vi "Send Write.vi"(8 "error in":errorcluster, 10 "Write":bool, 11 "MBs":refnum<class "Modbus Master CR.lvclass">[](array[class])) -> (0 "error out":errorcluster, 3 "MBs out":refnum<class "Modbus Master CR.lvclass">[](array[class]))   [LabVIEW 2021, in "Modbus Master CR.lvclass"]
uses:
  Modbus Master CR.lvclass
  Modbus Master CR.lvclass/Modbus Master CR.ctl
  <vilib>/Utility/error.llb/Clear Errors.vi
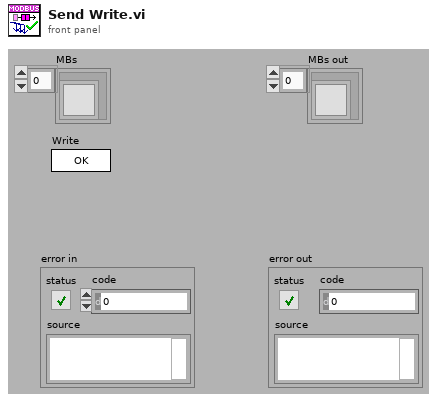
[diagram p1: front panel]
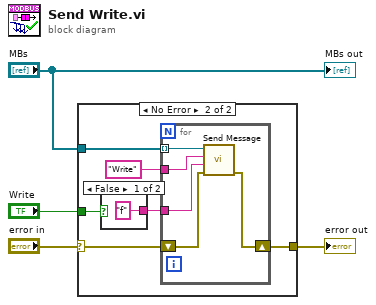
[diagram p0: block diagram]
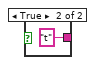
[diagram p3: hidden frame]
diagram:
  n1 = case shown="No Error" "error in" {
    selector: "error in" -> [w5 w11]
    tunnel: [w5 w8] -> w4
    tunnel: "MBs" -> [_ w6]
    tunnel: "Write" -> [_ w7]
    frame Error {
    }
    frame No Error {
      n2 = case shown="False" w7 {
        tunnel: ["f" ("Message") "t" ("Message")] -> w9
        frame False {
        }
        frame True {
        }
      }
      n3 = for {
        tunnel: "Write" ("Message") -> [w16]
        tunnel: w9 -> [w15]
        shift-right: [w14] -> w8
        shift-left: w11 -> [w13]
        tunnel: w6 -> [w12] mode=indexing
        n4 = call "Send Message.vi"("error in (no error)"=w13, "Message Data"=w15, "Message"=w16, "MB in"=w12) -> ("error out"=w14:errorcluster)  [unwired: 5 in, 2 out]
      }
    }
  }
  "error out" <- w4
  "MBs out" <- "MBs"
